vi "New SSLv23 Client Context.vi"(8 "error in (no error)":errorcluster, 11 "SSL-Lib":refnum<class "SSL-Lib.lvclass">) -> (0 "error out":errorcluster, 3 "SSL Client Context out":refnum<class "SSL Client Context.lvclass">)   [LabVIEW 2013, in "OpenSSL Socket.lvlib" / "SSL Client Context.lvclass"]
uses:
  SSL Client Context.lvclass
  SSL_Lib/SSL-Lib/SSL-Lib.lvclass
  SSL Context/SSL Context.lvclass/SSL Context.ctl
  SSL Context/Write SSL Context.vi
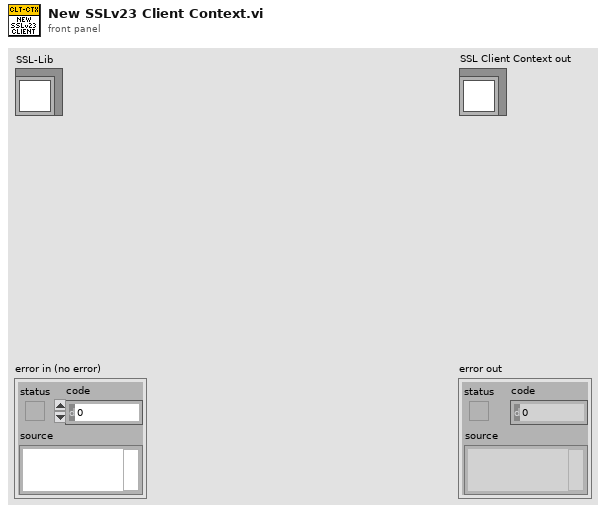
[diagram p1: front panel]
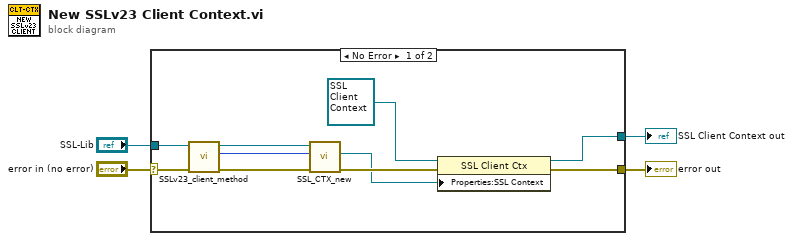
[diagram p0: block diagram]
diagram:
  n1 = case shown="No Error" "error in (no error)" {
    selector: "error in (no error)" -> [w11 w15]
    tunnel: [w5 w15] -> w3
    tunnel: [w6 _] -> w2
    tunnel: "SSL-Lib" -> [w10 _]
    frame No Error {
      n2 = call "SSLv23_client_method.vi"("error in (no error)"=w11, "SSL-Lib in"=w10) -> ("error out"=w12:errorcluster, "*SSL_Method"=w14:u64, "SSL-Lib out"=w13:refnum<class "SSL-Lib.lvclass">)  [unwired: 7 in]
      n3 = call "SSL_CTX_new.vi"("error in (no error)"=w12, "*SSL_Method"=w14, "SSL-Lib in"=w13) -> ("error out"=w9:errorcluster, "SSL-Context out"=w7:refnum<class "SSL-Context.lvclass">)  [unwired: 6 in, 1 out]
      n4 = property class="SSL Client Ctx"(reference=refnum<class "SSL Client Context.lvclass"> refnum ("OpenSSL Socket.lvlib:SSL Client Context.lvclass"), error in=w9, "Properties:SSL Context"=w7) -> (reference out=w6:refnum<class "SSL Client Context.lvclass">, error out=w5:errorcluster)
    }
    frame Error {
    }
  }
  "error out" <- w3
  "SSL Client Context out" <- w2
